vi "IsEnemy.vi"(1 "Black/White Turn (T/F)":bool, 2 "Column":i32, 3 "Row":i32, 4 "Board":i32[][](array[numeric])) -> (0 "Boolean":bool)   [LabVIEW 2014]
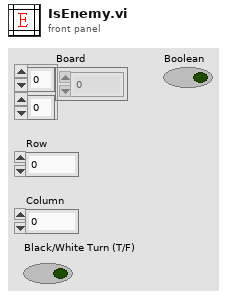
[diagram p1: front panel]
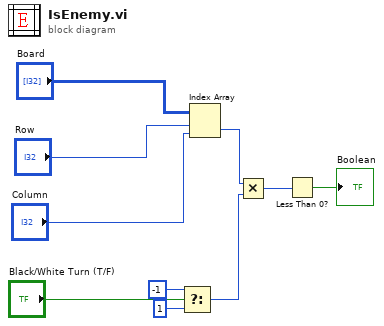
[diagram p0: block diagram]
diagram:
  n1 = Select(t=-1, s="Black/White Turn (T/F)", f=1) -> (s? t:f=w2:i32)
  n2 = Index Array(array="Board", index (row)="Row", index (col)="Column") -> (element=w4:i32)
  n3 = Multiply(x=w4, y=w2) -> (x*y=w1:i32)
  n4 = Less Than 0?(x=w1) -> (x < 0?=→"Boolean":bool)
